vi "Print List of Hardware.vi"   [LabVIEW 2016, in "Controller Actor.lvlib" / "Controller.lvclass"]
uses:
  <userlib>/Common Components/Controller/Controller.lvclass
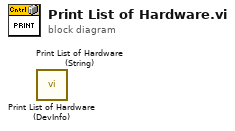
[diagram p0: block diagram]
diagram:
  n1 = call <userlib>:"Print List of Hardware (DevInfo).vi"() -> ()  [unwired: 11 in, 1 out]
  n2 = call <userlib>:"Print List of Hardware (String).vi"() -> ()  [unwired: 11 in, 1 out]
